vi "Populate Sub Menu.vi"(0 "Sample Type Sub Types":refnum<vi>, 7 "Base Path":path, 11 "Ring Text":string) -> (4 "Sample Type Sub Types (Dup)":refnum<vi>, 8 "Caption Text":string, 15 "Menu Items":string[](array[string]))   [LabVIEW 2016]
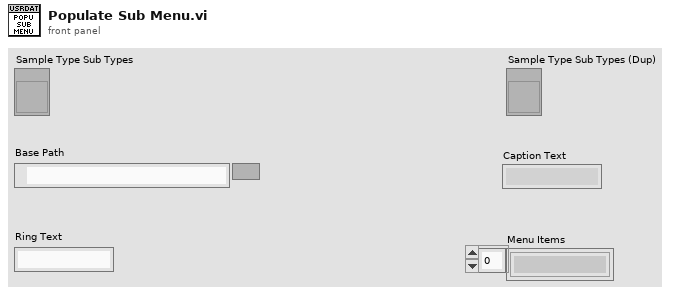
[diagram p1: front panel]
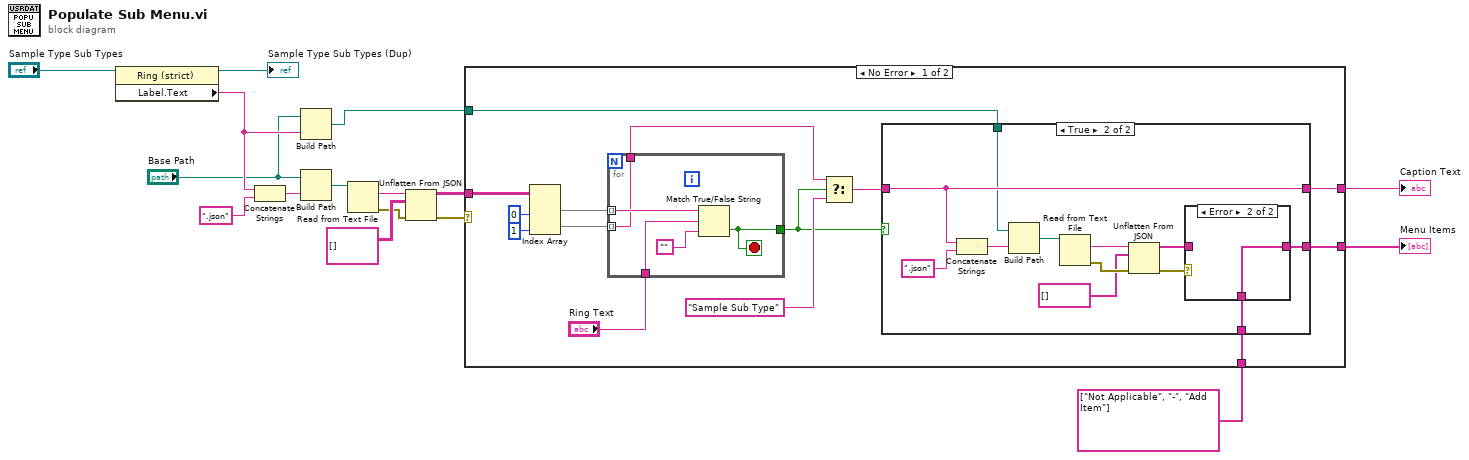
[diagram p0: block diagram]
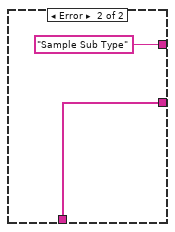
[diagram p4: hidden frame]
diagram:
  n1 = property class="Ring (strict)"(reference="Sample Type Sub Types") -> (reference out=→"Sample Type Sub Types (Dup)":refnum<vi>, "Label.Text"=w9:string)  [unwired: 1 in, 1 out]
  n2 = Concatenate Strings(w9, ".json") -> (w10:string)
  n3 = Build Path(base path="Base Path", name or relative path=w9) -> (appended path=w8:path)
  n4 = Build Path(base path="Base Path", name or relative path=w10) -> (appended path=w16:path)
  n5 = Read from Text File(file (use dialog)=w16) -> (text=w15:string, error out=w13:errorcluster)  [unwired: 3 in, 2 out]
  n6 = Unflatten From JSON(JSON string=w15, type and defaults=string[][] [], error in (no error)=w13) -> (value=w12:string[][], error out=w2:errorcluster)  [unwired: 4 in]
  n7 = case shown="No Error" w2 {
    tunnel: w12 -> [w29 _]
    tunnel: w8 -> [w21 _]
    tunnel: [w19 "Sample Sub Type"] -> w5
    tunnel: [w18 w53] -> w4
    tunnel: string[] ["Not Applicable", "-", "Add Item"] -> [w17 w53]
    frame No Error {
      n8 = Index Array(array=w29, index (col) #1=0 ("disabled index (col)"), index (col) #2=1 ("index (col)")) -> (element #1=w28:string[], element #2=w26:string[])  [unwired: 2 in]
      n9 = for {
        tunnel: w28 -> [w51] mode=indexing
        tunnel: w26 -> [w47] mode=indexing
        tunnel: "Ring Text" -> [w50]
        tunnel: [w48] -> w23
        tunnel: [w47] -> w25
        stop <- w48 stop-if-true
        n10 = Match True/False String(2:"", 3:w50, 4:w51) -> (0:w48:bool)  [unwired: 1 out]
      }
      n11 = Select(t=w25, s=w23, f="Sample Sub Type") -> (s? t:f=w22:string)
      n12 = case shown="True" w23 {
        tunnel: [w32 w43] -> w19
        tunnel: w22 -> [w32 w43]
        tunnel: w21 -> [_ w42]
        tunnel: w17 -> [w31 w34]
        tunnel: [w31 w33] -> w18
        frame False {
        }
        frame True {
          n13 = Concatenate Strings(w43, ".json") -> (w41:string)
          n14 = Build Path(base path=w42, name or relative path=w41) -> (appended path=w40:path)
          n15 = Read from Text File(file (use dialog)=w40) -> (text=w39:string, error out=w38:errorcluster)  [unwired: 3 in, 2 out]
          n16 = Unflatten From JSON(JSON string=w39, type and defaults=string[] [], error in (no error)=w38) -> (value=w35:string[], error out=w36:errorcluster)  [unwired: 4 in]
          n17 = case shown="Error" w36 {
            tunnel: w35 -> [w45 _]
            tunnel: [w45 w46] -> w33
            tunnel: w34 -> [_ w46]
            frame No Error {
            }
            frame Error {
            }
          }
        }
      }
    }
    frame Error {
    }
  }
  "Caption Text" <- w5
  "Menu Items" <- w4
